vi "Get Created Aliases.vi"(7 "jettl in":refnum<class "jettl.lvclass">, 10 "Addresses DVR":refnum<data-value>) -> (2 "Created Aliases":string[](array[string]), 5 "jettl out":refnum<class "jettl.lvclass">)   [LabVIEW 2021, in "jettl.lvlib" / "Addresses.lvlib" / "Addresses.lvclass"]
uses:
  Addresses.lvclass
  Addresses.lvclass/Addresses.ctl
  jettl/jettl.lvclass
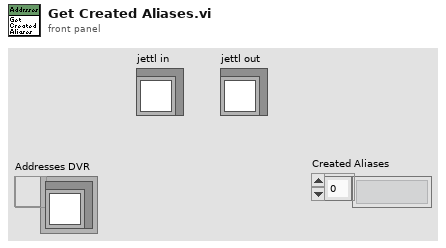
[diagram p1: front panel]
types:
  T1 = typedef "jettl.lvlib/Addresses.lvlib/Created.ctl" = map{string, refnum<class "Msg Type Strategy.lvclass">}
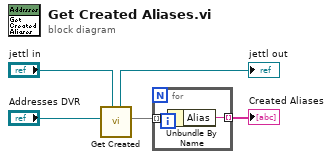
[diagram p0: block diagram]
diagram:
  n1 = call "Get Created.vi"("jettl in"="jettl in", "Addresses DVR"="Addresses DVR") -> ("Created"=w1:T1, "jettl out"=→"jettl out":refnum<class "jettl.lvclass">)  [unwired: 8 in]
  n2 = for {
    tunnel: [w6] -> w2 mode=indexing
    tunnel: w1 -> [w7] mode=indexing
    n3 = Unbundle By Name(w7) -> ("Alias"=w6:string)
  }
  "Created Aliases" <- w2
